vi "AppendFITSHeaderLine.vi"(4 "Entry Type":u16(ring) items=["String", "Numeric", "Boolean"], 5 "Comment":string, 6 "Entry #":dbl, 7 "error in (no error)":errorcluster, 8 "Element Value":string, 9 "Element Name":string, 10 "file path (dialog if empty)":path) -> (0 "error out":errorcluster)   [LabVIEW 2015]
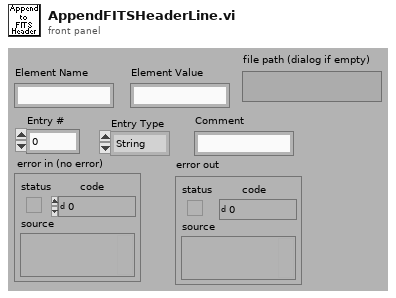
[diagram p1: front panel]
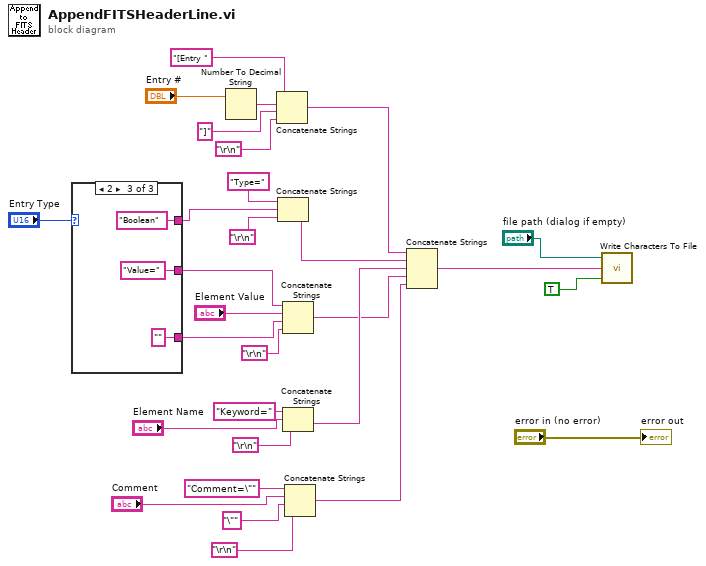
[diagram p0: block diagram]
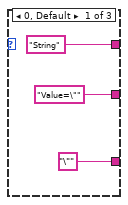
[diagram p2: hidden frame]
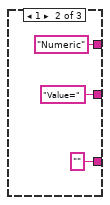
[diagram p3: hidden frame]
diagram:
  n1 = case shown="2" "Entry Type" {
    tunnel: ["String" ("string") "Numeric" ("string") "Boolean" ("string")] -> w19
    tunnel: ["Value=\"" ("string") "Value=" ("string") "Value=" ("string")] -> w13
    tunnel: ["\"" ("string") "" ("string") "" ("string")] -> w12
    frame 0, Default {
    }
    frame 1 {
    }
    frame 2 {
    }
  }
  n2 = Number To Decimal String(number="Entry #") -> (decimal integer string=w25:string)  [unwired: 1 in]
  n3 = Concatenate Strings("[Entry " ("string"), w25, "]" ("string"), "\r\n") -> (w10:string)
  n4 = Concatenate Strings("Type=" ("string"), w19, "\r\n") -> (w9:string)
  n5 = Concatenate Strings(w13, "Element Value", w12, "\r\n") -> (w7:string)
  n6 = Concatenate Strings("Keyword=" ("string"), "Element Name", "\r\n") -> (w8:string)
  n7 = Concatenate Strings("Comment=\"" ("string"), "Comment", "\"" ("string"), "\r\n") -> (w1:string)
  n8 = Concatenate Strings(w10, w9, w8, w7, w1) -> (w6:string)
  n9 = call <vilib>:"Write Characters To File.vi"("append to file? (new file:F)"=TRUE, "character string"=w6, "file path (dialog if empty)"="file path (dialog if empty)") -> ()  [unwired: 2 in, 1 out]
  "error out" <- "error in (no error)"
